vi "Vacuum Test - Step 2.vi"(7 "Step":i32, 8 "error in":errorcluster, 9 "Test Results In":T9, 10 "PAS In":T8 caption="Gas", 11 "Test Configuration":T1) -> (0 "error out":errorcluster, 1 "Test Results Out":T9, 2 "PAS Out":T8 caption="Gas", 3 "Test Configuration Out":T1)   [LabVIEW 2015]
uses:
  CAN Communication/PAS/Typedefs/Session Handle.ctl
  CAN Communication/PAS/PAS.lvclass
  Controls/Test Results.ctl
  Controls/Step Result.ctl
  Controls/Test Configuration.ctl
  Controls/Vacuum Test.ctl
  Controls/Test Timing.ctl
  Controls/Vaccum Thresholds.ctl
  Controls/Helium Test.ctl
  Controls/Helium Thresholds.ctl
  Controls/Functional Test.ctl
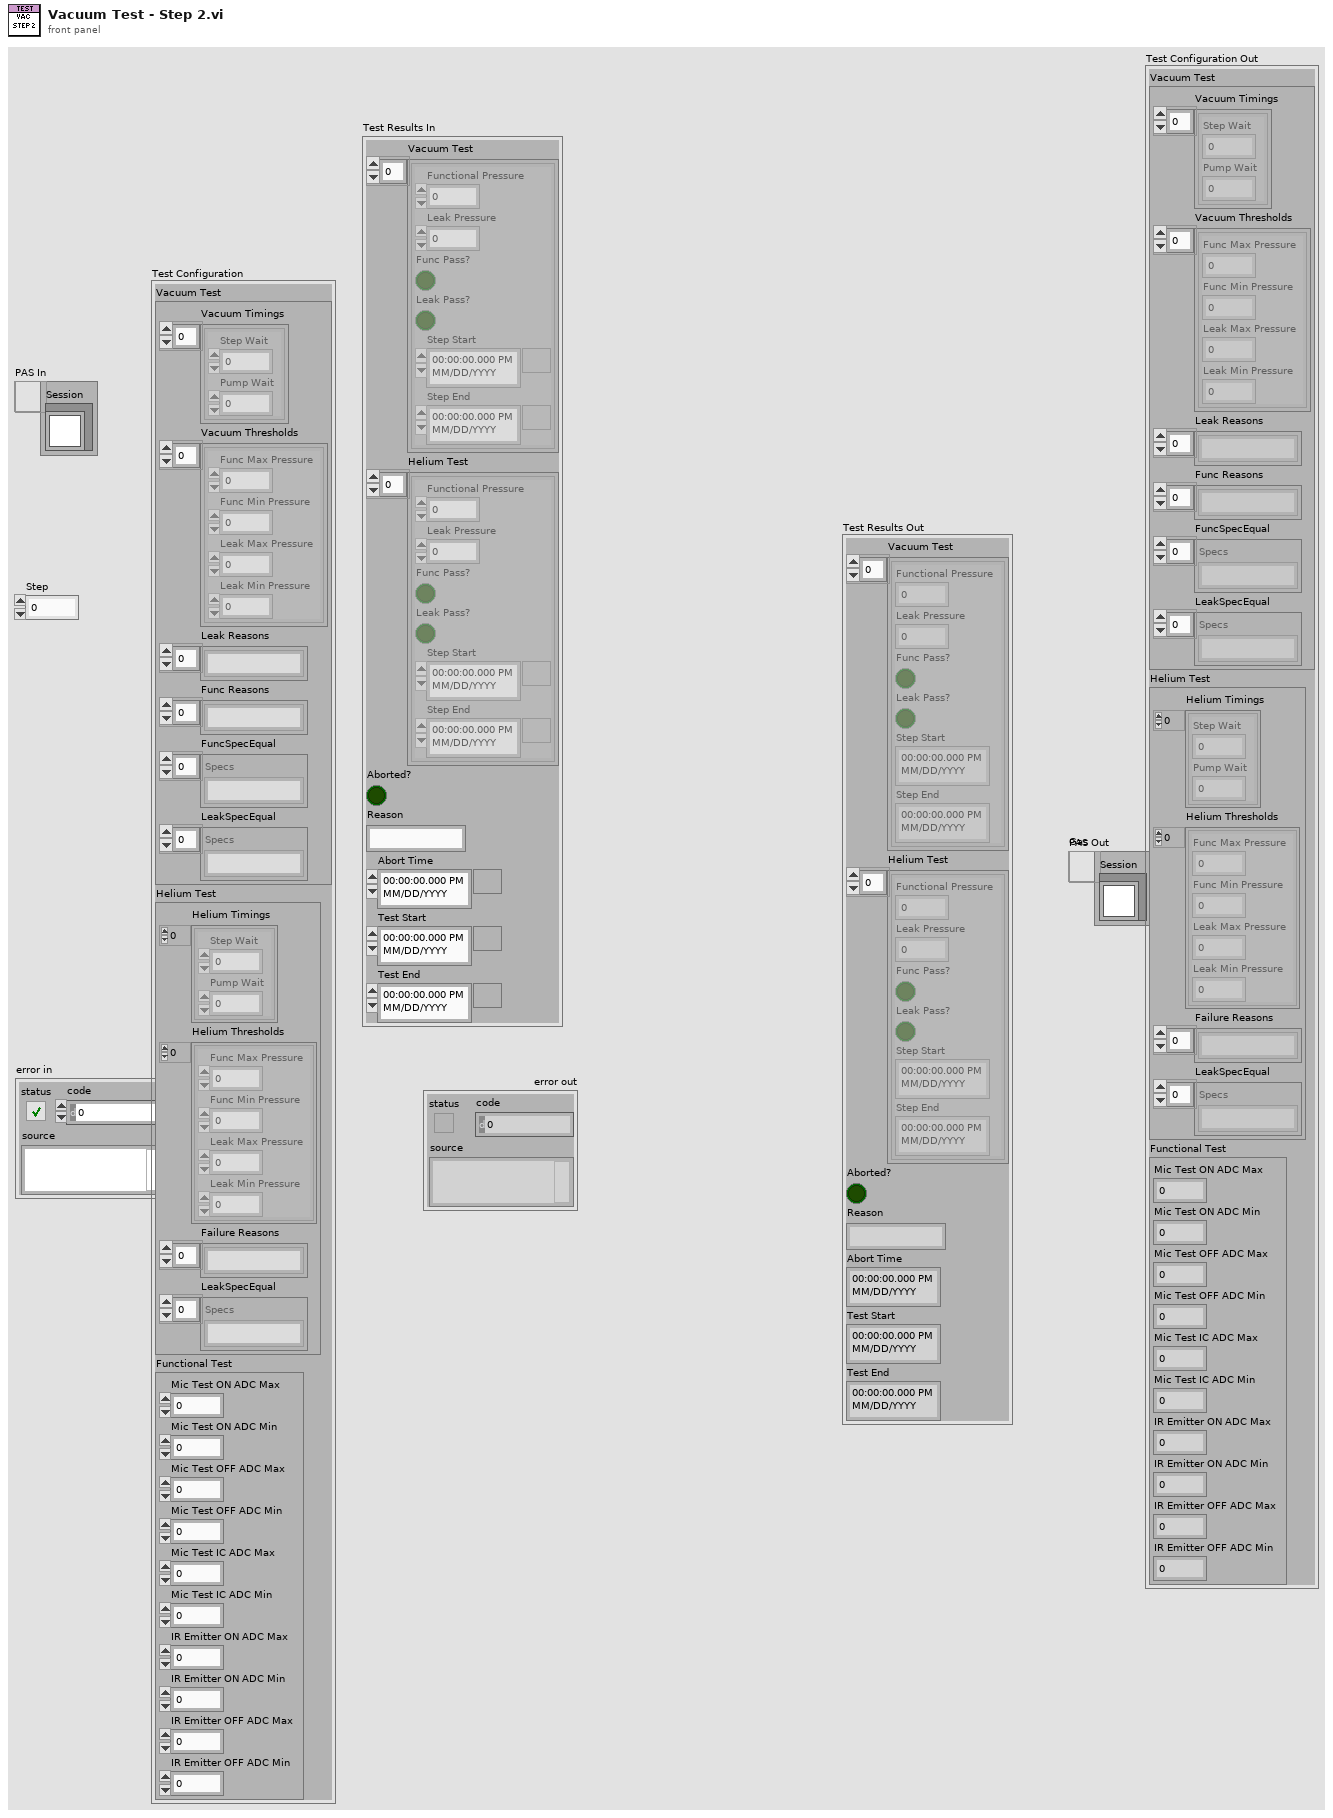
[diagram p1: front panel]
types:
  T1 = typedef "Test Configuration.ctl" = cluster{"Vacuum Test":T2, "Helium Test":T5, "Functional Test":T7}
  T2 = typedef "Vacuum Test.ctl" = cluster{"Vacuum Timings":T3[], "Vacuum Thresholds":T4[], "Leak Reasons":string[], "Func Reasons":string[], "FuncSpecEqual":string[], "LeakSpecEqual":string[]}
  T3 = typedef "Test Timing.ctl" = cluster{"Step Wait":dbl, "Pump Wait":dbl}
  T4 = typedef "Vaccum Thresholds.ctl" = cluster{"Func Max Pressure":dbl, "Func Min Pressure":dbl, "Leak Max Pressure":dbl, "Leak Min Pressure":dbl}
  T5 = typedef "Helium Test.ctl" = cluster{"Helium Timings":T3[], "Helium Thresholds":T6[], "Failure Reasons":string[], "LeakSpecEqual":string[]}
  T6 = typedef "Helium Thresholds.ctl" = cluster{"Func Max Pressure":dbl, "Func Min Pressure":dbl, "Leak Max Pressure":dbl, "Leak Min Pressure":dbl}
  T7 = typedef "Functional Test.ctl" = cluster{"Mic Test ON ADC Max":dbl, "Mic Test ON ADC Min":dbl, "Mic Test OFF ADC Max":dbl, "Mic Test OFF ADC Min":dbl, "Mic Test IC ADC Max":dbl, "Mic Test IC ADC Min":dbl, "IR Emitter ON ADC Max":dbl, "IR Emitter ON ADC Min":dbl, "IR Emitter OFF ADC Max":dbl, "IR Emitter OFF ADC Min":dbl}
  T8 = typedef "PAS.lvclass/Session Handle.ctl" = refnum<data-value>
  T9 = typedef "Test Results.ctl" = cluster{"Vacuum Test":T10[], "Helium Test":T10[], "Aborted?":bool, "Reason":string, "Abort Time":timestamp, "Test Start":timestamp, "Test End":timestamp}
  T10 = typedef "Step Result.ctl" = cluster{"Functional Pressure":dbl, "Leak Pressure":dbl, "Func Pass?":bool, "Leak Pass?":bool, "Step Start":timestamp, "Step End":timestamp}
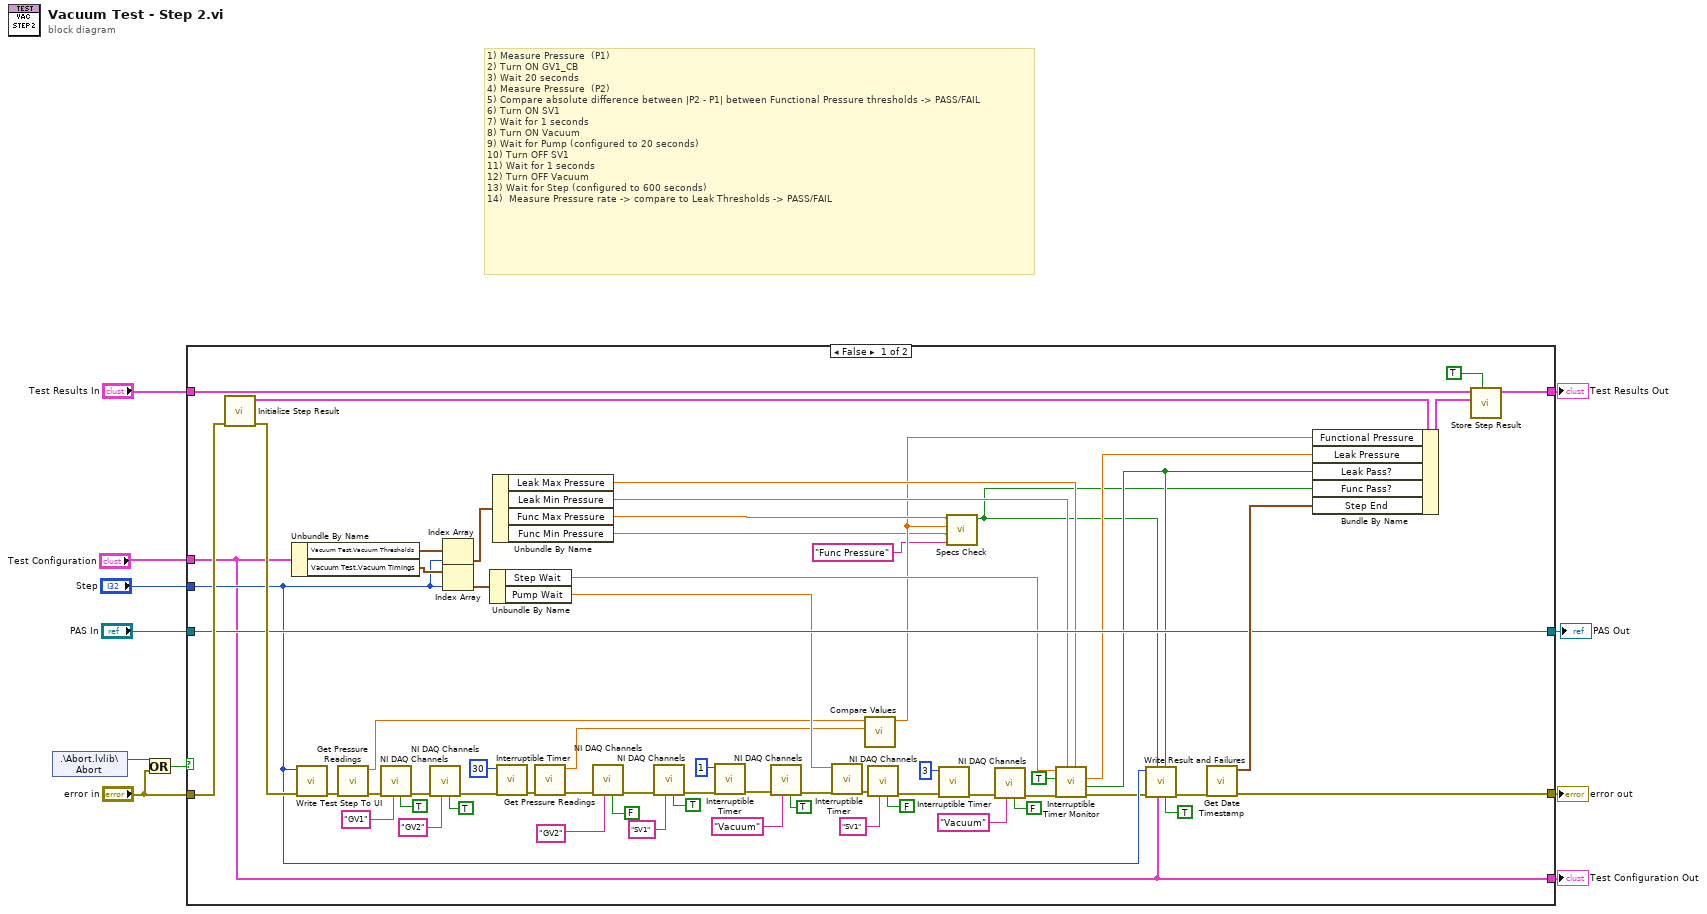
[diagram p0: block diagram]
diagram:
  # "1) Measure Pressure  (P1)\n2) Turn ON GV1_CB\n3) Wait 20 seconds\n4) Measure Pressure  (P2)\n5) Compare absolute difference between |P2 - P1| between Functional Pressure thresholds -> PASS/FAIL\n6) Turn ON SV1\n7) Wait for 1 seconds\n8) Turn ON Vacuum\n9) Wait for Pump (configured to 20 seconds)\n10) Turn OFF SV1\n11) Wait for 1 seconds\n12) Turn OFF Vacuum\n13) Wait for Step (configured to 600 seconds)\n14)  Measure Pressure rate -> compare to Leak Thresholds -> PASS/FAIL"
  n1 = shared-variable ".\\Abort.lvlib\\Abort"() -> (w10:bool)  [unwired: 1 in, 1 out]
  n2 = Or(x=w10, y="error in") -> (x .or. y?=w9:bool)
  n3 = case shown="False" w9 {
    tunnel: "error in" -> [w75 w78]
    tunnel: "Test Results In" -> [w72 w79]
    tunnel: [w73 w79] -> w7
    tunnel: [w25 w78] -> w6
    tunnel: "Test Configuration" -> [w52 w77]
    tunnel: "Step" -> [w60 _]
    tunnel: [w52 w77] -> w1
    tunnel: [w65 w76] -> w3
    tunnel: "PAS In" -> [w65 w76]
    frame False {
      n4 = call "Initialize Step Result.vi"("error in (no error)"=w75) -> ("error out"=w74:errorcluster, "New Step Result"=w71:T10)  [unwired: 8 in, 1 out]
      n5 = Unbundle By Name(w52) -> ("Vacuum Test.Vacuum Thresholds"=w68:T4[], "Vacuum Test.Vacuum Timings"=w67:T3[])
      n6 = call "Write Test Step To UI.vi"("error in (no error)"=w74, "Step"=w60) -> ("error out"=w51:errorcluster)  [unwired: 9 in]
      n7 = call "Get Pressure Readings.vi"("error in (no error)"=w51) -> ("error out"=w50:errorcluster, "NI-DAQ Pressure"=w42:dbl)  [unwired: 7 in, 2 out]
      n8 = call "NI DAQ Channels.vi"("Control"=TRUE ("State"), "Channel"="GV1", "error in (no error)"=w50) -> ("error out"=w40:errorcluster)  [unwired: 7 in, 1 out]
      n9 = call "NI DAQ Channels.vi"("Control"=TRUE ("State"), "Channel"="GV2", "error in (no error)"=w40) -> ("error out"=w38:errorcluster)  [unwired: 7 in, 1 out]
      n10 = Index Array(array=w68, index=w60) -> (element=w62:T4)
      n11 = Index Array(array=w67, index=w60) -> (element=w66:T3)
      n12 = Unbundle By Name(w66) -> ("Step Wait"=w33:dbl, "Pump Wait"=w63:dbl)
      n13 = Unbundle By Name(w62) -> ("Leak Max Pressure"=w30:dbl, "Leak Min Pressure"=w31:dbl, "Func Max Pressure"=w15:dbl, "Func Min Pressure"=w13:dbl)
      n14 = call "Interruptible Timer.vi"("error in (no error)"=w38, "Wait (s)"=30) -> ("error out"=w49:errorcluster)  [unwired: 7 in, 2 out]
      n15 = call "Get Pressure Readings.vi"("error in (no error)"=w49) -> ("error out"=w37:errorcluster, "NI-DAQ Pressure"=w41:dbl)  [unwired: 7 in, 2 out]
      n16 = call "NI DAQ Channels.vi"("Control"=FALSE ("State"), "Channel"="GV2", "error in (no error)"=w37) -> ("error out"=w36:errorcluster)  [unwired: 7 in, 1 out]
      n17 = call "NI DAQ Channels.vi"("Control"=TRUE ("State"), "Channel"="SV1", "error in (no error)"=w36) -> ("error out"=w45:errorcluster)  [unwired: 7 in, 1 out]
      n18 = call "Interruptible Timer.vi"("error in (no error)"=w45, "Wait (s)"=1) -> ("error out"=w46:errorcluster)  [unwired: 7 in, 2 out]
      n19 = call "NI DAQ Channels.vi"("Control"=TRUE ("State"), "Channel"="Vacuum", "error in (no error)"=w46) -> ("error out"=w44:errorcluster)  [unwired: 7 in, 1 out]
      n20 = call "Interruptible Timer.vi"("error in (no error)"=w44, "Wait (s)"=w63) -> ("error out"=w43:errorcluster)  [unwired: 7 in, 2 out]
      n21 = call "Compare Values.vi"("P2"=w41, "P1"=w42) -> ("Abs Diff"=w14:dbl)  [unwired: 9 in]
      n22 = call "NI DAQ Channels.vi"("Control"=FALSE ("State"), "Channel"="SV1", "error in (no error)"=w43) -> ("error out"=w56:errorcluster)  [unwired: 7 in, 1 out]
      n23 = call "Interruptible Timer.vi"("error in (no error)"=w56, "Wait (s)"=3) -> ("error out"=w53:errorcluster)  [unwired: 7 in, 2 out]
      n24 = call "Specs Check.vi"("parameter"="Func Pressure", "lower limit"=w13, "x"=w14, "upper limit"=w15) -> ("In Range?"=w16:bool)  [unwired: 6 in, 1 out]
      n25 = call "NI DAQ Channels.vi"("Control"=FALSE ("State"), "Channel"="Vacuum", "error in (no error)"=w53) -> ("error out"=w34:errorcluster)  [unwired: 7 in, 1 out]
      n26 = call "Interruptible Timer Monitor.vi"("Max"=w30, "Min"=w31, "error in (no error)"=w34, "Update UI?"=TRUE, "Wait (s)"=w33) -> ("error out"=w27:errorcluster, "In Range?"=w28:bool, "Leak Rate"=w29:dbl)  [unwired: 2 in, 2 out]
      n27 = call "Write Result and Failures.vi"("Vacuum?"=TRUE, "Leak"=w28, "Test Configuration"=w52, "Func"=w16, "error in (no error)"=w27, "Step"=w60) -> ("error out"=w26:errorcluster)  [unwired: 5 in]
      n28 = call "Get Date Timestamp.vi"("error in (no error)"=w26) -> ("error out"=w25:errorcluster, "current time"=w69:timestamp)  [unwired: 9 in]
      n29 = Bundle By Name(cluster=w71, "Functional Pressure"=w14, "Leak Pressure"=w29, "Leak Pass?"=w28, "Func Pass?"=w16, "Step End"=w69) -> (w70:T10)
      n30 = call "Store Step Result.vi"("Vacuum?"=TRUE, "Step Result"=w70, "Test Results In"=w72) -> ("Test Results Out"=w73:T9)  [unwired: 8 in]
    }
    frame True {
    }
  }
  "error out" <- w6
  "Test Results Out" <- w7
  "PAS Out" <- w3
  "Test Configuration Out" <- w1
